vi "dll.midi_connect_input.vi"(8 "error in (no error)":errorcluster, 10 "device_index":i32, 11 "LabVIEW-MIDI-XPLAT in":refnum<class "midi in.lvclass">) -> (0 "error out":errorcluster, 2 "Return":i32, 3 "LabVIEW-MIDI-XPLAT out":refnum<class "midi in.lvclass">)   [LabVIEW 2020, in "midi in.lvclass"]
uses:
  midi in.lvclass
  midi in.lvclass/midi in.ctl
  shared/midi shared.lvlib
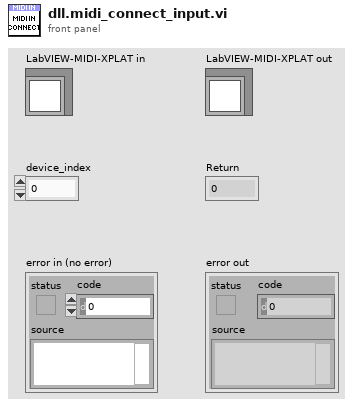
[diagram p1: front panel]
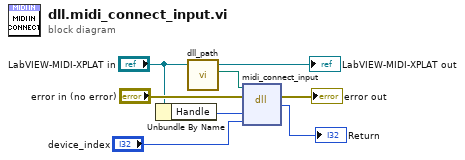
[diagram p0: block diagram]
diagram:
  n1 = Unbundle By Name("LabVIEW-MIDI-XPLAT in") -> ("Handle"=w4:i32)
  n2 = call "dll_path.vi"() -> ("dll"=w1:path)  [unwired: 11 in]
  n3 = dll-call lib="C:/code/LabVIEW-MIDI-XPLAT/dist/TomMIDIllan_*.*" fn="midi_connect_input"(path in=w1, error in="error in (no error)", "handle"=w4, "device_index"="device_index") -> (error out=→"error out":errorcluster, "Return"=→"Return":i32)  [unwired: 3 in, 1 out]
  "LabVIEW-MIDI-XPLAT out" <- "LabVIEW-MIDI-XPLAT in"
